vi "Get IND560 Scale Data.vi"(11 "VISA Refnum in":refnum<visa-resource-name>) -> (0 "error out":errorcluster, 1 "Displayed Net Wt.":dbl, 2 "Displayed Gross Wt.":dbl, 3 "VISA Refnum out":refnum<visa-resource-name>, 5 "IND560 Scale Data":string[][](array[string]))   [LabVIEW 2016]
panel:
  in  "Standard Runtime":string="CALLBACK wt0101 wt0102\nREAD ws0105 pt0101\n"
  out "read buffer":string
  in  "Login":string="USER admin\nUSER admin\nCONTOUT\nCTIMER 100\nCALLBACK wt0101 wt0102\nREAD ws0105"
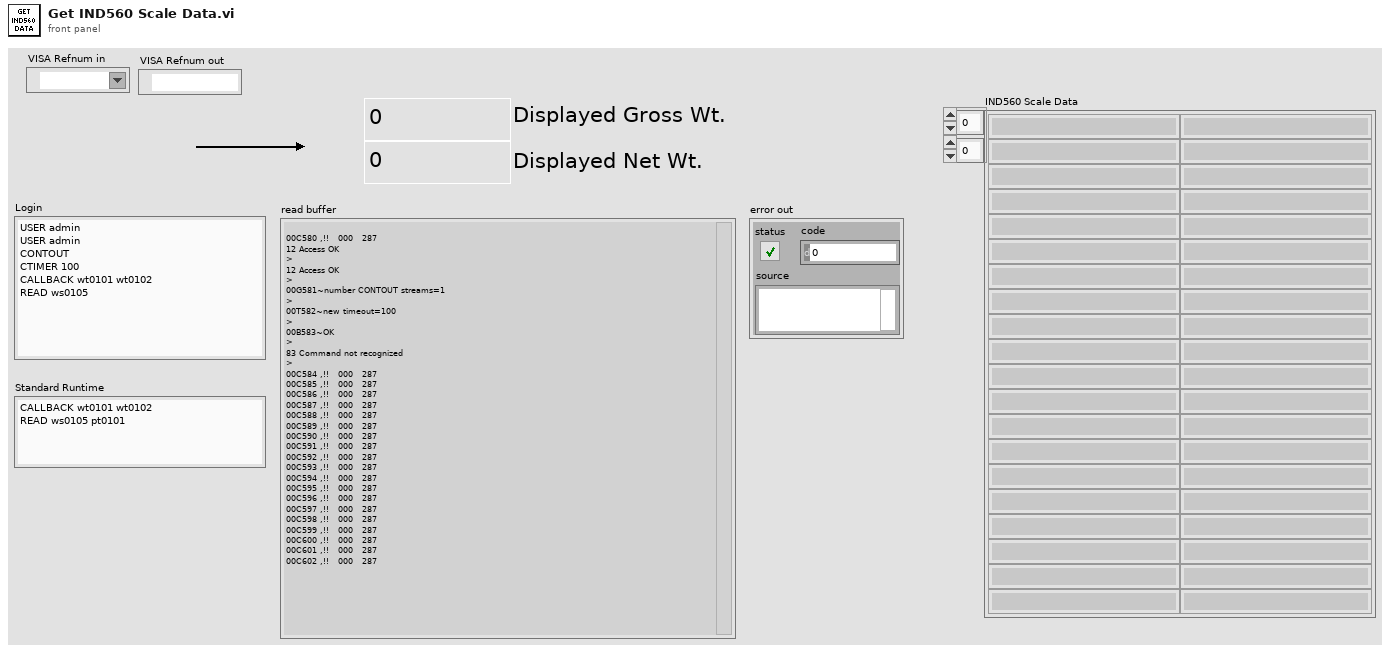
[diagram p1: front panel]
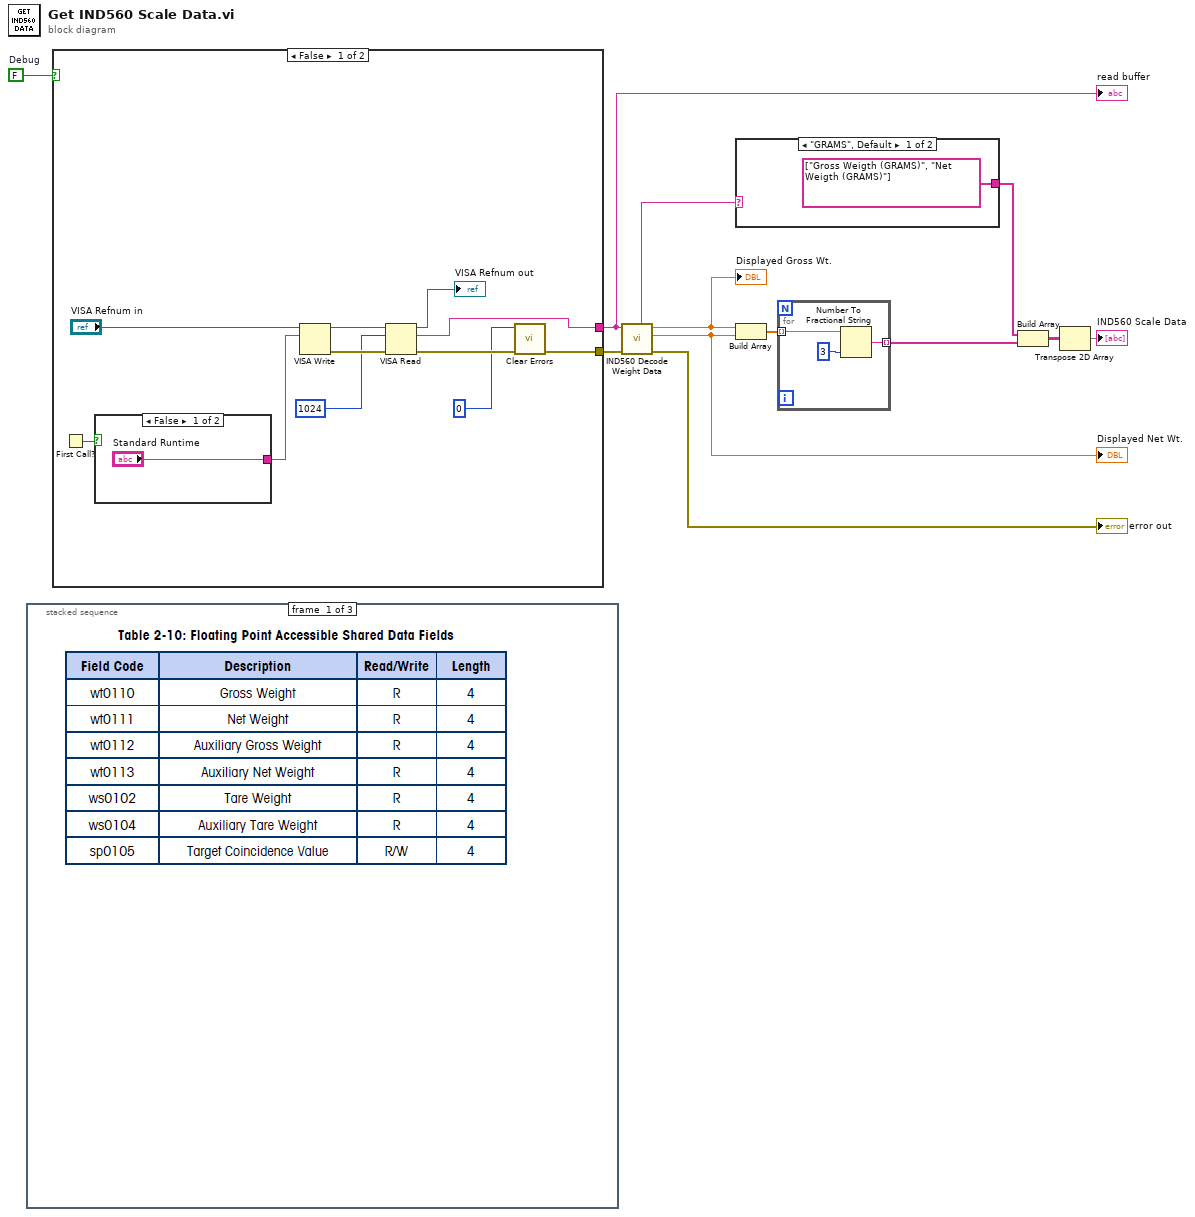
[diagram p0: block diagram]
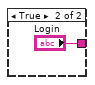
[diagram p2: hidden frame]
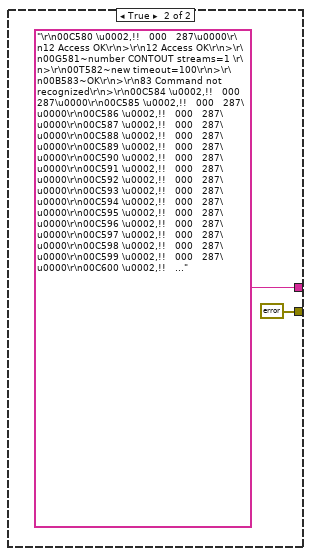
[diagram p3: hidden frame]
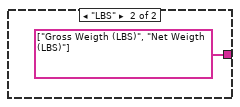
[diagram p4: hidden frame]
diagram:
  w1 = FALSE  # Debug
  n1 = stacked-sequence {
    frame #0 {
    }
    frame #1 {
    }
    frame #2 {
    }
  }
  n2 = case shown="False" w1 {
    tunnel: [w17 "\r\n00C580 \u0002,!!   000   287\u0000\r\n12 Access OK\r\n>\r\n12 Access OK\r\n>\r\n00G581~number CONTOUT streams=1 \r\n>\r\n00T582~new timeout=100\r\n>\r\n00B583~OK\r\n>\r\n83 Command not recognized\r\n>\r\n00C584 \u0002,!!   000   287\u0000\r\n00C585 \u0002,!!   000   287\u0000\r\n00C586 \u0002,!!   000   287\u0000\r\n00C587 \u0002,!!   000   287\u0000\r\n00C588 \u0002,!!   000   287\u0000\r\n00C589 \u0002,!!   000   287\u0000\r\n00C590 \u0002,!!   000   287\u0000\r\n00C591 \u0002,!!   000   287\u0000\r\n00C592 \u0002,!!   000   287\u0000\r\n00C593 \u0002,!!   000   287\u0000\r\n00C594 \u0002,!!   000   287\u0000\r\n00C595 \u0002,!!   000   287\u0000\r\n00C596 \u0002,!!   000   287\u0000\r\n00C597 \u0002,!!   000   287\u0000\r\n00C598 \u0002,!!   000   287\u0000\r\n00C599 \u0002,!!   000   287\u0000\r\n00C600 \u0002,!!   ..." ("read buffer")] -> w5
    tunnel: [w16 errorcluster {"status"=FALSE, "code"=0, "source"=""} ("error out")] -> w4
    frame False {
      n3 = First Call?() -> (First Call?: T/F=w15:bool)
      n4 = case shown="False" w15 {
        tunnel: ["Standard Runtime" "Login"] -> w20
        frame False {
        }
        frame True {
        }
      }
      n5 = VISA Write(VISA resource name="VISA Refnum in", write buffer=w20) -> (VISA resource name out=w22:refnum<visa-resource-name>, error out=w23:errorcluster)  [unwired: 1 in, 1 out]
      n6 = VISA Read(VISA resource name=w22, byte count=u32 1024 ("return count"), error in (no error)=w23) -> (VISA resource name out=→"VISA Refnum out":refnum<visa-resource-name>, read buffer=w17:string, error out=w18:errorcluster)  [unwired: 1 out]
      n7 = call <vilib>:"Clear Errors.vi"("error in (no error)"=w18, "specific error code to clear (0: all)"=0) -> ("error out"=w16:errorcluster)  [unwired: 4 in, 1 out]
    }
    frame True {
    }
  }
  "read buffer" <- w5
  n8 = call "IND560 Decode Weight Data.vi"("Error In"=w4, "read buffer"=w5) -> ("Error Out"=→"error out":errorcluster, "Displayed Net Wt."=w7:dbl, "Displayed Gross Wt."=w6:dbl, "Units"=w2:string)  [unwired: 6 in]
  "Displayed Net Wt." <- w7
  "Displayed Gross Wt." <- w6
  n9 = case shown="\"GRAMS\", Default" w2 {
    tunnel: [string[] ["Gross Weigth (GRAMS)", "Net Weigth (GRAMS)"] string[] ["Gross Weigth (LBS)", "Net Weigth (LBS)"]] -> w11
    frame "GRAMS", Default {
    }
    frame "LBS" {
    }
  }
  n10 = Build Array(w6, w7) -> (w9:dbl[])
  n11 = for {
    tunnel: w9 -> [w31] mode=indexing
    tunnel: [w30] -> w12 mode=indexing
    n12 = Number To Fractional String(number=w31, precision (6)=i16 3) -> (F-format string=w30:string)  [unwired: 2 in]
  }
  n13 = Build Array(w11, w12) -> (w10:string[][])
  n14 = Transpose 2D Array(2D array=w10) -> (transposed array=→"IND560 Scale Data":string[][])
